vi "Read Waveform Measurement (Standard).vi"(0 "VISA resource name":refnum<visa-resource-name>, 5 "Source (1: Channel 1)":u16(ring)=1 items=["Channel 1"=1, "Channel 2"=2, "Channel 3"=3, "Channel 4"=4], 9 "Measurement (0: Vpp)":u16(ring) items=["Vpp", "Vmax", "Vmin", "Vamp", "Vtop", "Vbase", "Vavg", "Mean", "Vrms", "Crms", "FOV", "FPRE", "ROV", "RPRE", "Period", "Freq", "+Wid", "-Wid", "Rise Time", "Fall Time", "Bwid", "+Duty", "-Duty"], 11 "error in (no error)":errorcluster) -> (4 "VISA resource name out":refnum<visa-resource-name>, 6 "Value":dbl, 15 "error out":errorcluster)   [LabVIEW 2021, in "Siglent SDS 1000 2000 Series.lvlib"]
doc: "Returns a the result of the requested measurement. Note that not all parameters are available on all scopes! (The VI will return an \"unresolved parsing error\" if an unsupported measurement is requested)\n\nThe measurements that you can select in this VI do not require arguments such as reference levels, slopes, etc; for parameters that require \"arguments\" configure them on the scope, and readout the result with the VI \"Read Px Measurement.vi\"\n\nNote that most \"horizontal\" parameters (e.g. parameters that return a time or frequency) are multi-valued. For these parameters, the last occurence is returned, as opposed to the average value over the entire sweep."
uses:
  <instrlib>/Siglent SDS 1000 2000 Series/Siglent SDS 1000 2000 Series.lvlib
panel:
  # "Note for functions with a *: The last measured value is returned by these functions, and not the average value  over the sweep. See VI help for more information."
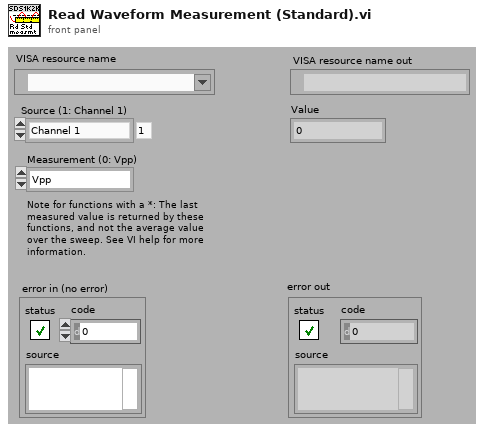
[diagram p1: front panel]
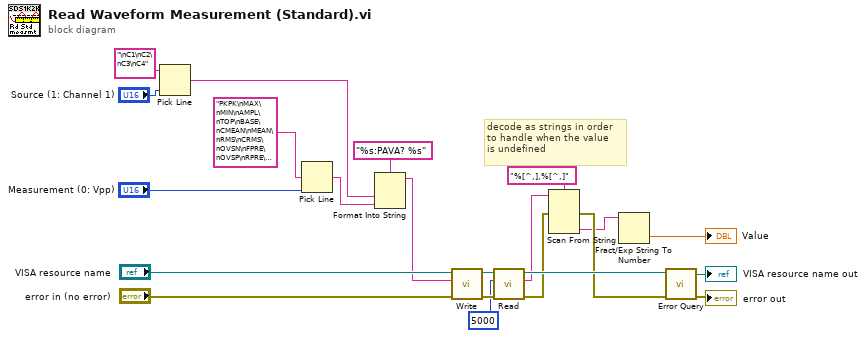
[diagram p0: block diagram]
diagram:
  # "decode as strings in order \nto handle when the value\nis undefined"
  n1 = Pick Line(multi-line string="\nC1\nC2\nC3\nC4", line index="Source (1: Channel 1)") -> (output string=w1:string)  [unwired: 1 in]
  n2 = Pick Line(multi-line string="PKPK\nMAX\nMIN\nAMPL\nTOP\nBASE\nCMEAN\nMEAN\nRMS\nCRMS\nOVSN\nFPRE\nOVSP\nRPRE\nPER\nFREQ\nPWID\nNWID\nRISE\nFALL\nWID\nDUTY\nNDUTY", line index="Measurement (0: Vpp)") -> (output string=w18:string)  [unwired: 1 in]
  n3 = Format Into String(format string="%s:PAVA? %s", w1, w18) -> (resulting string=w10:string)  [unwired: 2 in, 1 out]
  n4 = call <instrlib>:"Write.vi"("error in (no error)"="error in (no error)", "Write Buffer"=w10, "VISA resource name"="VISA resource name") -> ("error out"=w15:errorcluster, "VISA resource name out"=w16:refnum<visa-resource-name>)  [unwired: 6 in, 1 out]
  n5 = call <instrlib>:"Read.vi"("error in (no error)"=w15, "Byte Count"=u32 5000, "VISA resource name"=w16) -> ("error out"=w6:errorcluster, "Read Buffer"=w7:string, "VISA resource name out"=w13:refnum<visa-resource-name>)  [unwired: 5 in, 1 out]
  n6 = Scan From String(format string="%[^,],%[^,]", input string=w7, error in=w6) -> (error out=w5:errorcluster, output 2=w3:string)  [unwired: 4 in, 2 out]
  n7 = Fract/Exp String To Number(string=w3) -> (number=→"Value":dbl)  [unwired: 3 in, 1 out]
  n8 = call <instrlib>:"Error Query.vi"("error in (no error)"=w5, "VISA resource name"=w13) -> ("error out"=→"error out":errorcluster, "VISA resource name out"=→"VISA resource name out":refnum<visa-resource-name>)  [unwired: 6 in, 2 out]
